vi "Main.vi"() -> ()   [LabVIEW 2018]
uses:
  Digit--control.ctl
  Temp Coef--control.ctl
  Multiplier--control.ctl
  Tolerance--control.ctl
  States--control.ctl
  Data--control.ctl
  E Series Reader/Data--control.ctl
  E Series Reader/E Series Reader.lvlib
panel:
  out "vn":dbl format="%#_2p"
  in  "Tol sel":T1 caption="Tolerance"
  out "TC Color":u32(colorbox) caption="TC"
  out "Tol Color":u32(colorbox) caption="Tol"
  out "M Color":u32(colorbox) caption="M"
  out "3D Color":u32(colorbox) caption="3D"
  out "2D Color":u32(colorbox) caption="2D"
  out "1D Color":u32(colorbox) caption="1D"
  in  "D3 sel":T2 caption="Digit 3"
  in  "D2 sel":T2 caption="Digit 2"
  in  "M sel":T3 caption="Multiplier"
  in  "TC sel":T4 caption="Temp Coef"
  in  "D1 sel":T2 caption="Digit 1"
  in  "Numero de bandas":u8=4 min=4 max=6 step=1
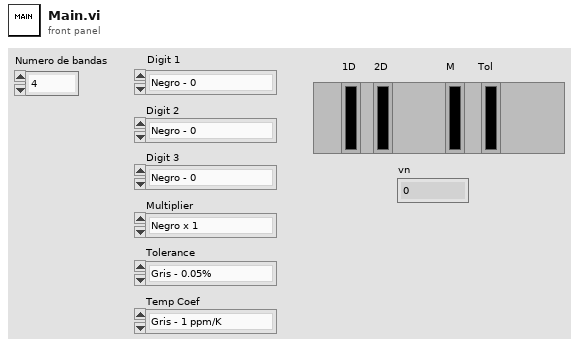
[diagram p1: front panel]
types:
  T1 = typedef "Tolerance--control.ctl" = enum16{"Gris - 0.05%", "Violeta - 0.1%", "Azul - 0.25%", "Verde - 0.5%", "Marron - 1%", "Rojo - 2%", "Oro - 5%", "Plata - 10%", "Ninguno - 20%"}
  T2 = typedef "Digit--control.ctl" = enum16{"Negro - 0", "Marron - 1", "Rojo - 2", "Naranja - 3", "Amarillo - 4", "Verde - 5", "Azul - 6", "Violeta - 7", "Gris - 8", "Blanco - 9"}
  T3 = typedef "Multiplier--control.ctl" = enum16{"Negro x 1", "Marron x 10", "Rojo x 100", "Naranja x 1K", "Amarillo x 10K", "Verde x 100K", " Azul x 1M", "Violeta x 10M ", "Oro x 0.1", "Plata x 0.01"}
  T4 = typedef "Temp Coef--control.ctl" = enum16{"Gris - 1 ppm/K", "Violeta - 5 ppm/K", "Azul - 10 ppm/K", "Verde - 20 ppm/K", "Amarillo - 25 ppm/K", "Naranja - 15 ppm/K", "Rojo - 50 ppm/K", "Marron - 100 ppm/K", "Negro - 250 ppm/K"}
  T5 = typedef "Data--control.ctl" = cluster{"D1 s Refn":refnum<vi>, "D2 s Refn":refnum<vi>, "D3 s Refn":refnum<vi>, "M s Reln":refnum<vi>, "Tol s Refn":refnum<vi>, "TC s Refn":refnum<vi>, "1D c Refn":refnum<vi>, "2D c Refn":refnum<vi>, "3D c Refn":refnum<vi>, "M c Refn":refnum<vi>, "Tol c Refn":refnum<vi>, "TC c Refn":refnum<vi>, "Data":T6, "Digit 1":T2, "Digit 2":T2, "Digit 3":T2, "Multiplier":T3, "Tolerance":T1, "Temp Coef":T4, "1D color":u32, "2D color":u32, "3D color":u32, "Mult":u32, "Tol":u32, "TC":u32}
  T6 = typedef "E Series Reader.lvlib/Data--control.ctl" = cluster{"E3 Series":u16[], "E6 Series ":u16[], "E12 Series":u16[], "E24 Series":u16[], "E48 Series":u16[], "E96 Series":u16[], "E192 Series":u16[]}
  T7 = typedef "States--control.ctl" = enum16{"Initialize", "Read E Series", "Get Color Number", "Read Parameters", "Organize Bands Colors", "Organize Bands Selectors", "Get Resistance Value", "Error", "Shutdown"}
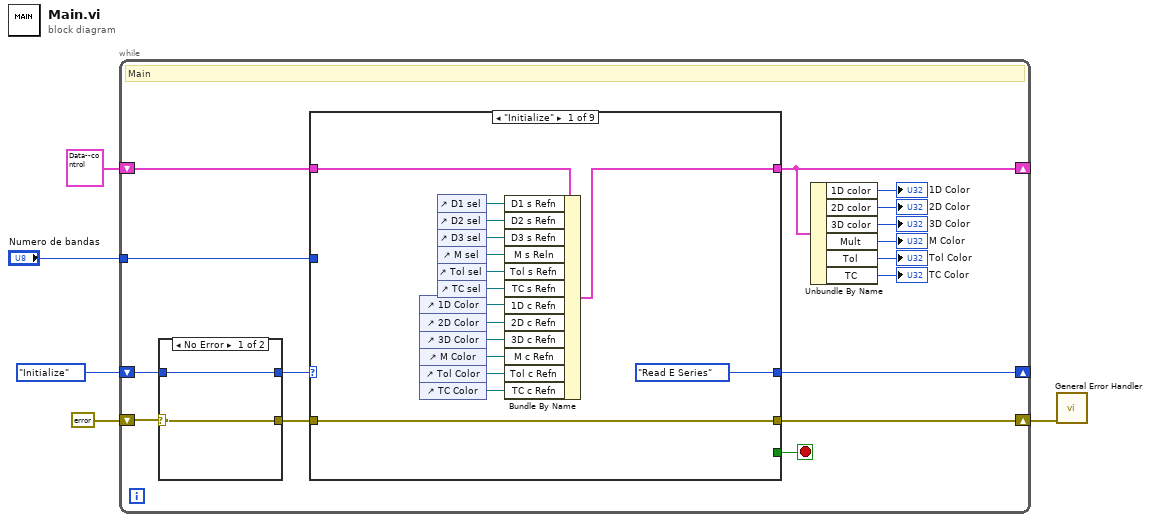
[diagram p0: block diagram]
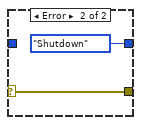
[diagram p2: hidden frame]
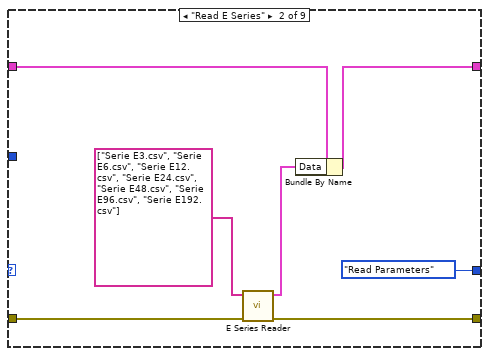
[diagram p3: hidden frame]
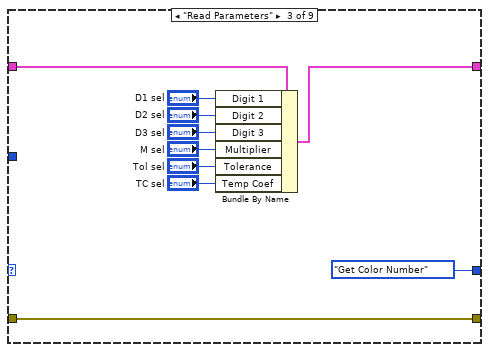
[diagram p4: hidden frame]
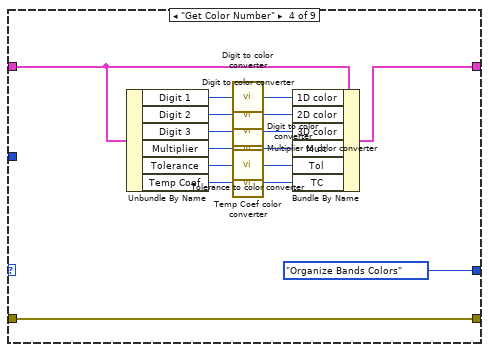
[diagram p5: hidden frame]
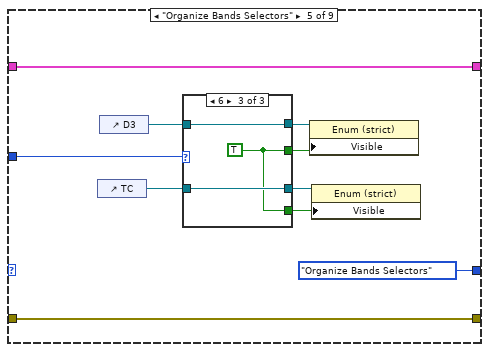
[diagram p6: hidden frame]
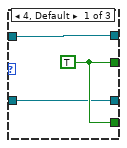
[diagram p7: hidden frame]
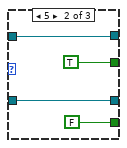
[diagram p8: hidden frame]
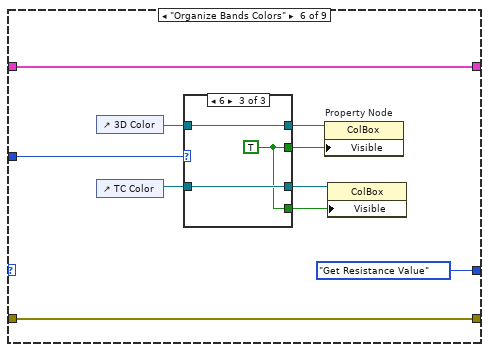
[diagram p9: hidden frame]
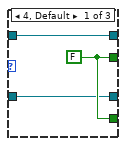
[diagram p10: hidden frame]
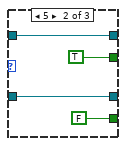
[diagram p11: hidden frame]
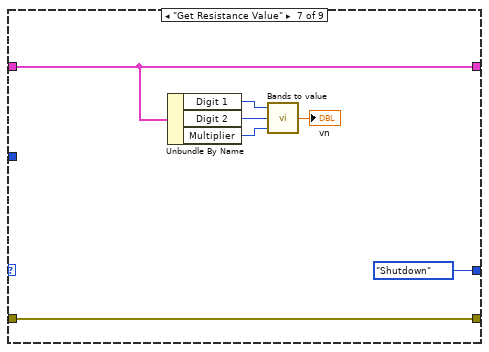
[diagram p12: hidden frame]
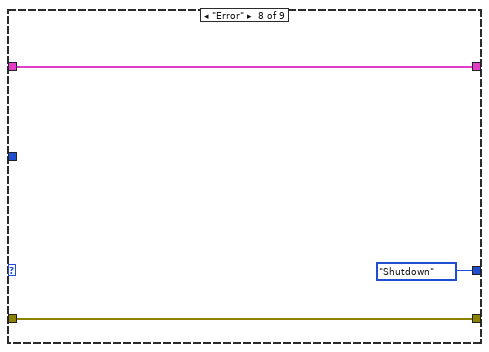
[diagram p13: hidden frame]
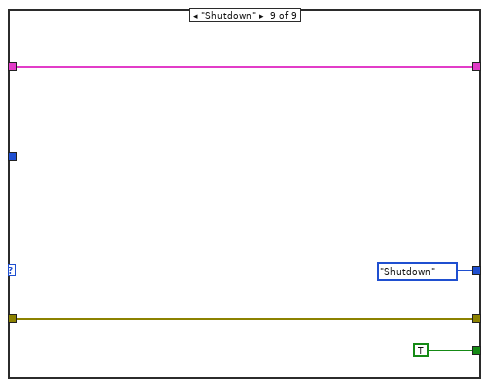
[diagram p14: hidden frame]
diagram:
  n1 = while {
    shift-right: [w17] -> _
    shift-left: States--control."Initialize" ("Enum") -> [w21]
    shift-right: [w13] -> w1
    shift-left: errorcluster {"status"=FALSE, "code"=0, "source"=""} ("error in") -> [w20]
    tunnel: "Numero de bandas" -> [w15]
    shift-right: [w12] -> _
    shift-left: T5 {"D1 s Refn"=refnum, "D2 s Refn"=refnum, "D3 s Refn"=refnum, "M s Reln"=refnum, "Tol s Refn"=refnum, "TC s Refn"=refnum, "1D c Refn"=refnum, "2D c Refn"=refnum, "3D c Refn"=refnum, "M c Refn"=refnum, "Tol c Refn"=refnum, "TC c Refn"=refnum, "Data"={"E3 Series"=[], "E6 Series "=[], "E12 Series"=[], "E24 Series"=[], "E48 Series"=[], "E96 Series"=[], "E192 Series"=[]}, "Digit 1"=enum."Negro - 0", "Digit 2"=enum."Negro - 0", "Digit 3"=enum."Negro - 0", "Multiplier"=enum."Negro x 1", "Tolerance"=enum."Gris - 0.05%", "Temp Coef"=enum."Gris - 1 ppm/K", "1D color"=0, "2D color"=0, "3D color"=0, "Mult"=0, "Tol"=0, "TC"=0} -> [w14]
    stop <- w16 stop-if-true
    # "Main"
    n2 = case shown="No Error" w20 {
      selector: w20 -> [w23 w25]
      tunnel: w21 -> [w22 _]
      tunnel: [w23 w25] -> w19
      tunnel: [w22 States--control."Shutdown" ("Enum")] -> w18
      frame No Error {
      }
      frame Error {
      }
    }
    n3 = case shown="\"Initialize\"" w18 {
      tunnel: w19 -> [w41 w46 w50 w60 w83 w103 w121 w122 w125]
      tunnel: [States--control."Read E Series" ("Enum") States--control."Read Parameters" ("Enum") States--control."Get Color Number" ("Enum") States--control."Organize Bands Colors" ("Enum") States--control."Organize Bands Selectors" ("Enum") States--control."Get Resistance Value" ("Enum") States--control."Shutdown" ("Enum") States--control."Shutdown" ("Enum") States--control."Shutdown" ("Enum")] -> w17
      tunnel: [_ _ _ _ _ _ _ _ TRUE] -> w16
      tunnel: w15 -> [_ _ _ _ w78 w98 _ _ _]
      tunnel: w14 -> [w39 w48 w58 w62 w84 w104 w120 w124 w128]
      tunnel: [w32 w47 w52 w61 w84 w104 w120 w124 w128] -> w12
      tunnel: [w41 w45 w50 w60 w83 w103 w121 w122 w125] -> w13
      frame "Initialize" {
        n4 = control-ref of="1D Color"() -> (w31:refnum<vi>)
        n5 = control-ref of="2D Color"() -> (w30:refnum<vi>)
        n6 = control-ref of="3D Color"() -> (w29:refnum<vi>)
        n7 = control-ref of="M Color"() -> (w28:refnum<vi>)
        n8 = control-ref of="Tol Color"() -> (w27:refnum<vi>)
        n9 = control-ref of="TC Color"() -> (w26:refnum<vi>)
        n10 = control-ref of="D1 sel"() -> (w38:refnum<vi>)
        n11 = control-ref of="D2 sel"() -> (w37:refnum<vi>)
        n12 = control-ref of="D3 sel"() -> (w36:refnum<vi>)
        n13 = control-ref of="M sel"() -> (w35:refnum<vi>)
        n14 = control-ref of="Tol sel"() -> (w34:refnum<vi>)
        n15 = control-ref of="TC sel"() -> (w33:refnum<vi>)
        n16 = Bundle By Name(cluster=w39, "D1 s Refn"=w38, "D2 s Refn"=w37, "D3 s Refn"=w36, "M s Reln"=w35, "Tol s Refn"=w34, "TC s Refn"=w33, "1D c Refn"=w31, "2D c Refn"=w30, "3D c Refn"=w29, "M c Refn"=w28, "Tol c Refn"=w27, "TC c Refn"=w26) -> (w32:T5)
      }
      frame "Read E Series" {
        n17 = call "E Series Reader.vi"("error in"=w46, "File name"=string[] ["Serie E3.csv", "Serie E6.csv", "Serie E12.csv", "Serie E24.csv", "Serie E48.csv", "Serie E96.csv", "Serie E192.csv"]) -> ("error out"=w45:errorcluster, "E Series"=w44:T6)  [unwired: 8 in]
        n18 = Bundle By Name(cluster=w48, "Data"=w44) -> (w47:T5)
      }
      frame "Read Parameters" {
        n19 = Bundle By Name(cluster=w58, "Digit 1"="D1 sel", "Digit 2"="D2 sel", "Digit 3"="D3 sel", "Multiplier"="M sel", "Tolerance"="Tol sel", "Temp Coef"="TC sel") -> (w52:T5)
      }
      frame "Get Color Number" {
        n20 = Unbundle By Name(w62) -> ("Digit 1"=w74:T2, "Digit 2"=w73:T2, "Digit 3"=w72:T2, "Multiplier"=w71:T3, "Tolerance"=w70:T1, "Temp Coef"=w69:T4)
        n21 = call "Digit to color converter.vi"("Digit"=w74) -> ("Digit color"=w68:u32)  [unwired: 4 in]
        n22 = call "Digit to color converter.vi"("Digit"=w73) -> ("Digit color"=w67:u32)  [unwired: 4 in]
        n23 = call "Digit to color converter.vi"("Digit"=w72) -> ("Digit color"=w66:u32)  [unwired: 4 in]
        n24 = call "Multiplier to color converter.vi"("Multiplier"=w71) -> ("Multiplier to color"=w65:u32)  [unwired: 4 in]
        n25 = call "Tolerance to color converter.vi"("Tolerance"=w70) -> ("Tolerance to  color"=w64:u32)  [unwired: 4 in]
        n26 = call "Temp Coef color converter.vi"("Temp Coef"=w69) -> ("Temp Coef to color"=w63:u32)  [unwired: 4 in]
        n27 = Bundle By Name(cluster=w62, "1D color"=w68, "2D color"=w67, "3D color"=w66, "Mult"=w65, "Tol"=w64, "TC"=w63) -> (w61:T5)
      }
      frame "Organize Bands Selectors" {
        n28 = control-ref of="TC"() -> (w81:refnum<vi>)
        n29 = control-ref of="D3"() -> (w82:refnum<vi>)
        n30 = case shown="6" w78 {
          tunnel: w82 -> [w86 w91 w94]
          tunnel: w81 -> [w85 w90 w93]
          tunnel: [w86 w91 w94] -> w80
          tunnel: [w85 w90 w93] -> w79
          tunnel: [w87 TRUE w92] -> w77
          tunnel: [w87 FALSE w92] -> w76
          frame 4, Default {
            w87 = TRUE
          }
          frame 5 {
          }
          frame 6 {
            w92 = TRUE
          }
        }
        n31 = property class="Enum (strict)"(reference=w80, "Visible"=w77) -> ()  [unwired: 1 in, 2 out]
        n32 = property class="Enum (strict)"(reference=w79, "Visible"=w76) -> ()  [unwired: 1 in, 2 out]
      }
      frame "Organize Bands Colors" {
        n33 = control-ref of="3D Color"() -> (w102:refnum<vi>)
        n34 = control-ref of="TC Color"() -> (w100:refnum<vi>)
        n35 = case shown="6" w98 {
          tunnel: w102 -> [w106 w111 w114]
          tunnel: [w106 w111 w114] -> w101
          tunnel: w100 -> [w105 w110 w113]
          tunnel: [w105 w110 w113] -> w99
          tunnel: [w107 TRUE w112] -> w97
          tunnel: [w107 FALSE w112] -> w96
          frame 4, Default {
            w107 = FALSE
          }
          frame 5 {
          }
          frame 6 {
            w112 = TRUE
          }
        }
        n36 = property on="Property Node" class="ColBox"(reference=w101, "Visible"=w97) -> ()  [unwired: 1 in, 2 out]
        n37 = property class="ColBox"(reference=w99, "Visible"=w96) -> ()  [unwired: 1 in, 2 out]
      }
      frame "Get Resistance Value" {
        n38 = Unbundle By Name(w120) -> ("Digit 1"=w118:T2, "Digit 2"=w117:T2, "Multiplier"=w116:T3)
        n39 = call "Bands to value.vi"("Multiplier"=w116, "Digit 2"=w117, "Digit"=w118) -> ("vn"=→"vn":dbl)  [unwired: 2 in]
      }
      frame "Error" {
      }
      frame "Shutdown" {
      }
    }
    n40 = Unbundle By Name(w12) -> ("1D color"=→"1D Color":u32, "2D color"=→"2D Color":u32, "3D color"=→"3D Color":u32, "Mult"=→"M Color":u32, "Tol"=→"Tol Color":u32, "TC"=→"TC Color":u32)
  }
  n41 = call <vilib>:"General Error Handler.vi"("error in (no error)"=w1) -> ()  [unwired: 10 in, 5 out]
